vi "CoreFileSaver.vi"(11 "Cluster":T1) -> ()   [LabVIEW 2024]
uses:
  #SaveFileEnum.ctl
  <vilib>/vision/Image Controls.llb/IMAQ Image.ctl
  vision/#QueueEnum.ctl
  GUI/#GuiEnum.ctl
  GUI/#GuiQueueElement.ctl
  Correlation/#CorrelationQueueElement.ctl
  Core/#CoreQueues.ctl
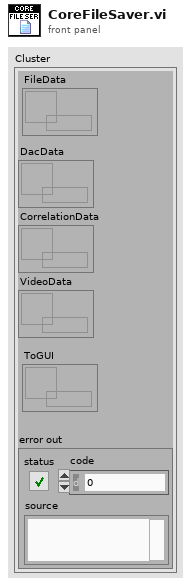
[diagram p1: front panel]
types:
  T1 = typedef "#CoreQueues.ctl" = cluster{"DacData":refnum<queue>, "CorrelationData":refnum<queue>, "VideoData":refnum<queue>, "error out":errorcluster, "ToGUI":refnum<queue>, "FileData":refnum<queue>}
  T2 = typedef "#SaveFileEnum.ctl" = enum16{"Idle", "Open", "Save", "Close"}
  T3 = enum16{"open", "open or create", "create or replace", "create", "open (read-only)"}
  T4 = typedef "#SaveFileParameters.ctl" = cluster{"StartSaveFile":bool, "TDMS file path":path}
  T5 = typedef "#CorrelationQueueElement.ctl" = cluster{"Enum":T6, "t0":timestamp, dbl[]}
  T6 = typedef "#QueueEnum.ctl" = enum16{"Ant", "Video"}
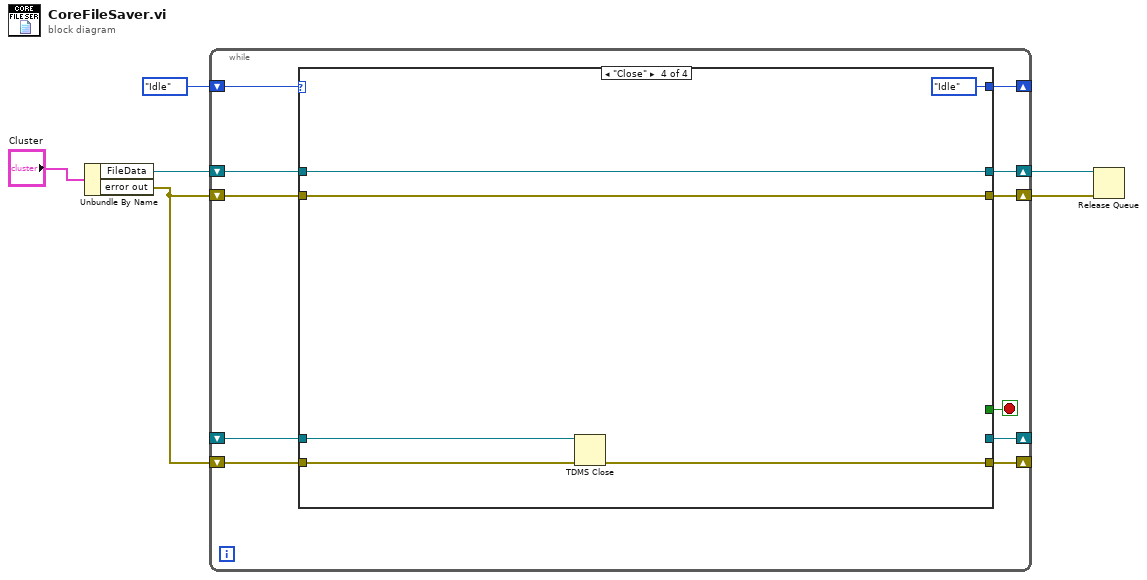
[diagram p0: block diagram]
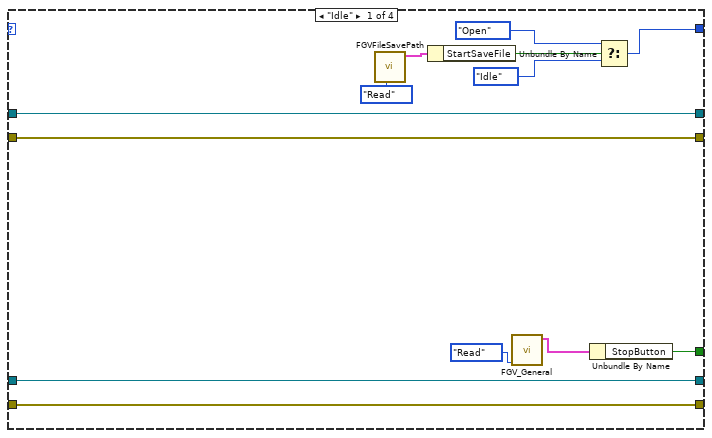
[diagram p2: hidden frame]
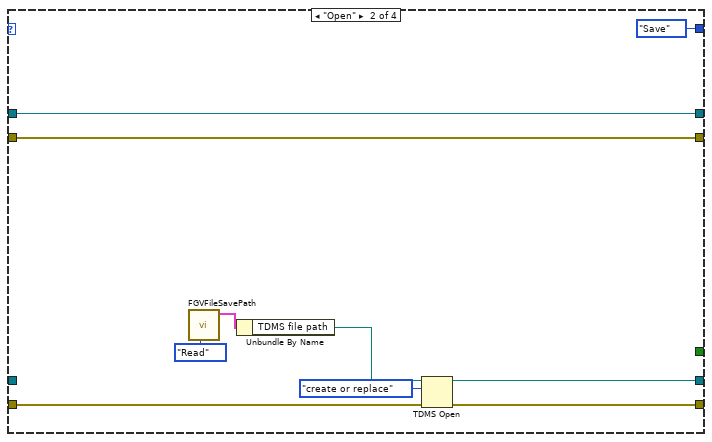
[diagram p3: hidden frame]
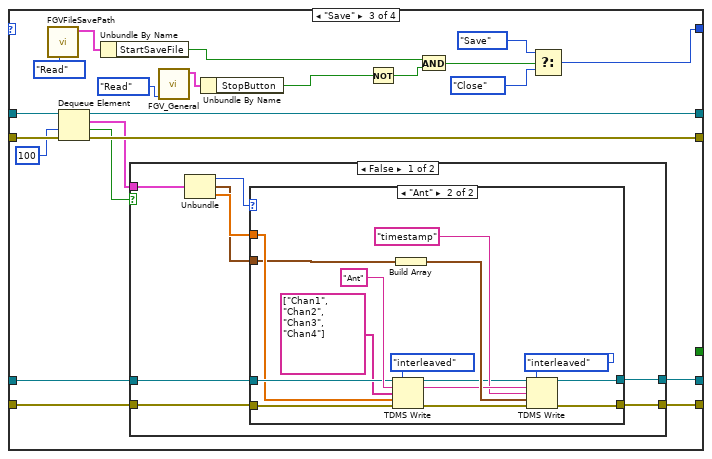
[diagram p4: hidden frame]
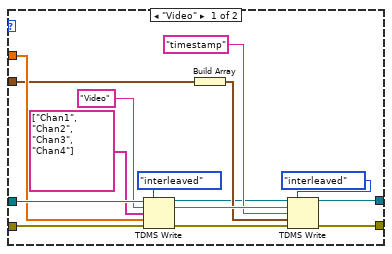
[diagram p5: hidden frame]
diagram:
  n1 = Unbundle By Name("Cluster") -> ("FileData"=w1:refnum<queue>, "error out"=w3:errorcluster)
  n2 = while {
    shift-right: [w15] -> w5
    shift-left: w1 -> [w17]
    shift-right: [w14] -> w6
    shift-left: w3 -> [w16]
    shift-right: [w13] -> _
    shift-left: _ -> [w10]
    shift-right: [w12] -> _
    shift-left: w3 -> [w11]
    shift-right: [w8] -> _
    shift-left: #SaveFileEnum."Idle" -> [w9]
    stop <- w7 stop-if-true
    n3 = case shown="\"Close\"" w9 {
      tunnel: w17 -> [w30 w37 w58 w105]
      tunnel: w16 -> [w29 w36 w56 w104]
      tunnel: [w30 w37 w57 w105] -> w15
      tunnel: [w29 w36 w55 w104] -> w14
      tunnel: [w26 w40 w60 _] -> w13
      tunnel: [w25 w39 w59 w106] -> w12
      tunnel: w11 -> [w25 w38 w62 w107]
      tunnel: w10 -> [w26 _ w61 w108]
      tunnel: [w23 #SaveFileEnum."Save" ("s? t:f") w41 #SaveFileEnum."Idle" ("s? t:f")] -> w8
      tunnel: [w18 _ _ _] -> w7
      frame "Idle" {
        n4 = call "FGVFileSavePath.vi"("Type"=enum16{"Read", "Write"}."Read") -> ("FileSaveParameters"=w27:T4)  [unwired: 10 in]
        n5 = Unbundle By Name(w27) -> ("StartSaveFile"=w24:bool)
        n6 = call "FGV_General.vi"("Type"=enum16{"Read", "Write"}."Read") -> ("GeneralIndicator"=w20:cluster{"StartButton":bool, "StopButton":bool})  [unwired: 10 in]
        n7 = Unbundle By Name(w20) -> ("StopButton"=w18:bool)
        n8 = Select(t=#SaveFileEnum."Open" ("s? t:f"), s=w24, f=#SaveFileEnum."Idle" ("s? t:f")) -> (s? t:f=w23:T2)
      }
      frame "Open" {
        n9 = call "FGVFileSavePath.vi"("Type"=enum16{"Read", "Write"}."Read") -> ("FileSaveParameters"=w34:T4)  [unwired: 10 in]
        n10 = Unbundle By Name(w34) -> ("TDMS file path"=w33:path)
        n11 = TDMS Open(8:w38, 10:T3."create or replace" ("operation (0:open)"), 11:w33) -> (0:w39:errorcluster, 3:w40:refnum<k34>)  [unwired: 4 in]
      }
      frame "Save" {
        n12 = call "FGVFileSavePath.vi"("Type"=enum16{"Read", "Write"}."Read") -> ("FileSaveParameters"=w50:T4)  [unwired: 10 in]
        n13 = Dequeue Element(queue=w58, timeout in ms (-1)=100, error in (no error)=w56) -> (queue out=w57:refnum<queue>, element=w52:T5, timed out?=w53:bool, error out=w55:errorcluster)
        n14 = Unbundle By Name(w50) -> ("StartSaveFile"=w43:bool)
        n15 = case shown="False" w53 {
          tunnel: w62 -> [w70 w101]
          tunnel: w61 -> [w69 w102]
          tunnel: [w68 w102] -> w60
          tunnel: [w67 w101] -> w59
          tunnel: w52 -> [w66 _]
          frame False {
            n16 = Unbundle(w66) -> ("Enum"=w65:T6, "t0"=w63:timestamp, w64:dbl[])
            n17 = case shown="\"Ant\"" w65 {
              tunnel: w70 -> [w85 w98]
              tunnel: w69 -> [w84 w99]
              tunnel: [w72 w90] -> w68
              tunnel: [w75 w87] -> w67
              tunnel: w64 -> [w82 w97]
              tunnel: w63 -> [w71 w86]
              frame "Video" {
                n18 = TDMS Write(0:w84, 1:enum16{"decimated", "interleaved"}."interleaved" ("data layout (0:decimated)"), 5:"Video" ("group name in (Untitled)"), 7:string[] ["Chan1", "Chan2", "Chan3", "Chan4"] ("channel name(s) in (Untitled)"), 9:w82, 11:w85) -> (4:w73:refnum<k34>, 6:w79:string, 15:w74:errorcluster)  [unwired: 1 out]
                n19 = Build Array(w71) -> (w78:timestamp[])
                n20 = TDMS Write(0:w73, 1:enum16{"decimated", "interleaved"}."interleaved" ("data layout (0:decimated)"), 5:w79, 7:"timestamp" ("channel name(s) in (Untitled)"), 9:w78, 11:w74) -> (4:w72:refnum<k34>, 15:w75:errorcluster)  [unwired: 2 out]
              }
              frame "Ant" {
                n21 = TDMS Write(0:w99, 1:enum16{"decimated", "interleaved"}."interleaved" ("data layout (0:decimated)"), 5:"Ant" ("group name in (Untitled)"), 7:string[] ["Chan1", "Chan2", "Chan3", "Chan4"] ("channel name(s) in (Untitled)"), 9:w97, 11:w98) -> (4:w89:refnum<k34>, 6:w93:string, 15:w88:errorcluster)  [unwired: 1 out]
                n22 = Build Array(w86) -> (w94:timestamp[])
                n23 = TDMS Write(0:w89, 1:enum16{"decimated", "interleaved"}."interleaved" ("data layout (0:decimated)"), 5:w93, 7:"timestamp" ("channel name(s) in (Untitled)"), 9:w94, 11:w88) -> (4:w90:refnum<k34>, 15:w87:errorcluster)  [unwired: 2 out]
              }
            }
          }
          frame True {
          }
        }
        n24 = call "FGV_General.vi"("Type"=enum16{"Read", "Write"}."Read") -> ("GeneralIndicator"=w47:cluster{"StartButton":bool, "StopButton":bool})  [unwired: 10 in]
        n25 = Unbundle By Name(w47) -> ("StopButton"=w44:bool)
        n26 = Not(x=w44) -> (.not. x?=w45:bool)
        n27 = And(x=w43, y=w45) -> (x .and. y?=w42:bool)
        n28 = Select(t=#SaveFileEnum."Save" ("s? t:f"), s=w42, f=#SaveFileEnum."Close" ("s? t:f")) -> (s? t:f=w41:T2)
      }
      frame "Close" {
        n29 = TDMS Close(8:w107, 11:w108) -> (0:w106:errorcluster)  [unwired: 1 out]
      }
    }
  }
  n30 = Release Queue(queue=w5, error in (no error)=w6) -> ()  [unwired: 1 in, 3 out]
